vi "Comp-HorarioSeg.vi"(1 "Lower limit":string, 2 "Upper limit":string) -> (0 "In Range?":bool)   [LabVIEW 2018]
panel:
  out "S string":string
  out "M string":string
  out "H string":string
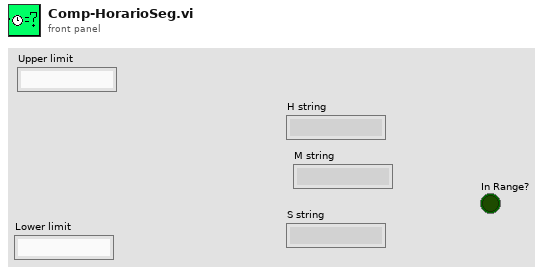
[diagram p1: front panel]
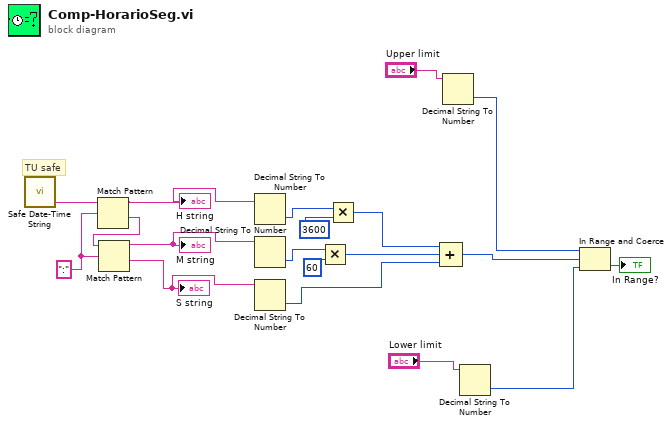
[diagram p0: block diagram]
diagram:
  w15 = ":" ("search string/char (-)")
  # "TU safe"
  n1 = call "Safe Date-Time String.vi"() -> ("Safe time string"=w1:string)  [unwired: 3 in, 1 out]
  n2 = Match Pattern(string=w1, regular expression=w15) -> (before substring=w14:string, after substring=w16:string)  [unwired: 1 in, 2 out]
  "H string" <- w14
  n3 = Match Pattern(string=w16, regular expression=w15) -> (before substring=w13:string, after substring=w12:string)  [unwired: 1 in, 2 out]
  "M string" <- w13
  "S string" <- w12
  n4 = Decimal String To Number(string=w14) -> (number=w8:i32)  [unwired: 2 in, 1 out]
  n5 = Decimal String To Number(string=w13) -> (number=w9:i32)  [unwired: 2 in, 1 out]
  n6 = Decimal String To Number(string=w12) -> (number=w5:i32)  [unwired: 2 in, 1 out]
  n7 = Multiply(x=w9, y=60 ("offset past number")) -> (x*y=w6:i32)
  n8 = Multiply(x=w8, y=3600 ("offset past number")) -> (x*y=w7:i32)
  n9 = Compound Arithmetic op=ADD(w7, w6, w5) -> (w17:i32)
  n10 = Decimal String To Number(string="Upper limit") -> (number=w4:i32)  [unwired: 2 in, 1 out]
  n11 = Decimal String To Number(string="Lower limit") -> (number=w2:i32)  [unwired: 2 in, 1 out]
  n12 = In Range and Coerce(upper limit=w4, x=w17, lower limit=w2) -> (In Range?=→"In Range?":bool)  [unwired: 1 out]
